vi "SubVI_Verificar_angulo_encontrado.vi"(1 "menor que, dê errado (graus)":dbl, 2 "maior que, dê errado (graus)":dbl, 3 "Angulo encontrado em Rad":dbl) -> (0 "Resultado(Rad)":dbl)   [LabVIEW 2017]
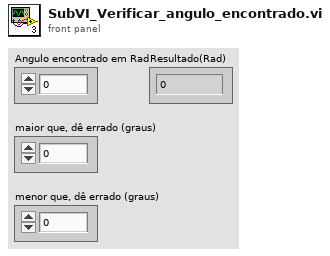
[diagram p1: front panel]
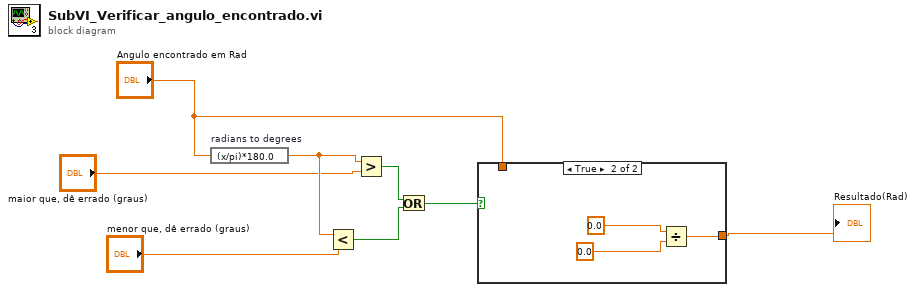
[diagram p0: block diagram]
diagram:
  n1 = expression code="(x/pi)*180.0" "radians to degrees"("Angulo encontrado em Rad") -> (w2:dbl)
  n2 = Less?(x=w2, y="menor que, dê errado (graus)") -> (x < y?=w5:bool)
  n3 = Greater?(x=w2, y="maior que, dê errado (graus)") -> (0:w4:bool)
  n4 = Or(x=w4, y=w5) -> (x .or. y?=w6:bool)
  n5 = case shown="True" w6 {
    tunnel: [w9 w10] -> w7
    tunnel: "Angulo encontrado em Rad" -> [w9 _]
    frame False {
    }
    frame True {
      n6 = Divide(x=0.0, y=0.0) -> (x/y=w10:dbl)
    }
  }
  "Resultado(Rad)" <- w7
